vi "Menu.vi"() -> ()   [LabVIEW 2021]
panel:
  out "error out":errorcluster
  in  "error in":errorcluster
  out "String":string
  in  "Exit":bool
  out "Access":bool
  in  "Cluster":T1
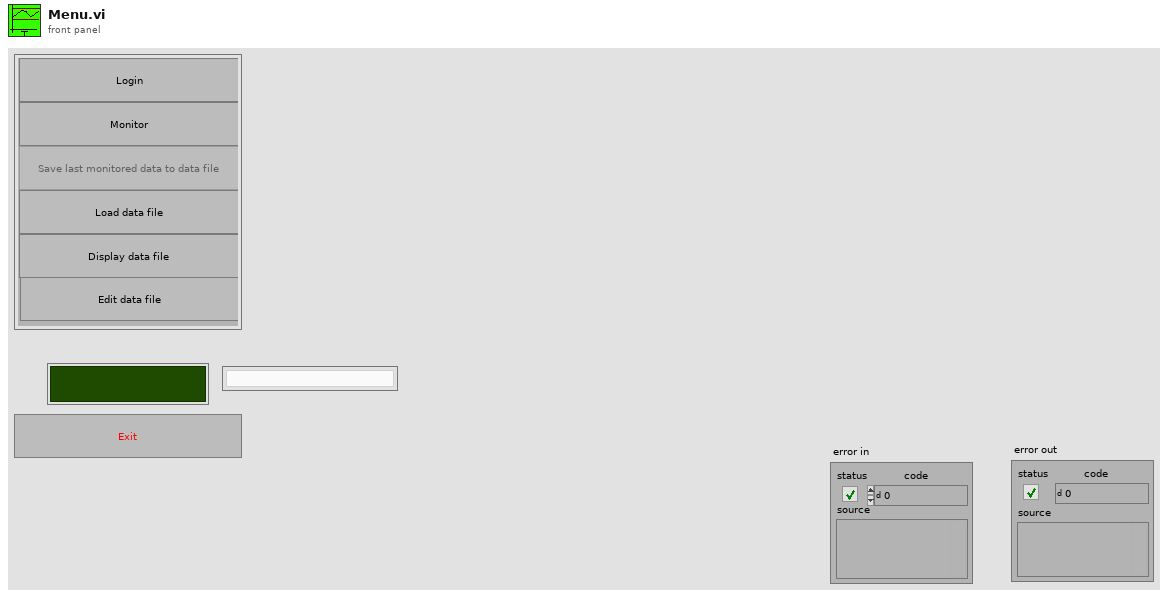
[diagram p1: front panel]
types:
  T1 = cluster{"Login button":bool, "Monitor button":bool, "Save data button":bool, "Load data button":bool, "Display data button":bool, "Edit Data File":bool}
  T2 = enum8{"Enabled", "Disabled", "Disabled and Grayed Out"}
  T3 = cluster{"User Name output":string, "Time/Date":timestamp, "Datos Finales":cluster{"Temp.Max":dbl, "Temp.Actual":dbl, "Temp.Min":dbl}[]}
  T4 = cluster{"User Name":string, "Time/Date":timestamp, "Datos Finales":cluster{"Temp.Max":dbl, "Temp.Actual":dbl, "Temp.Min":dbl}[]}
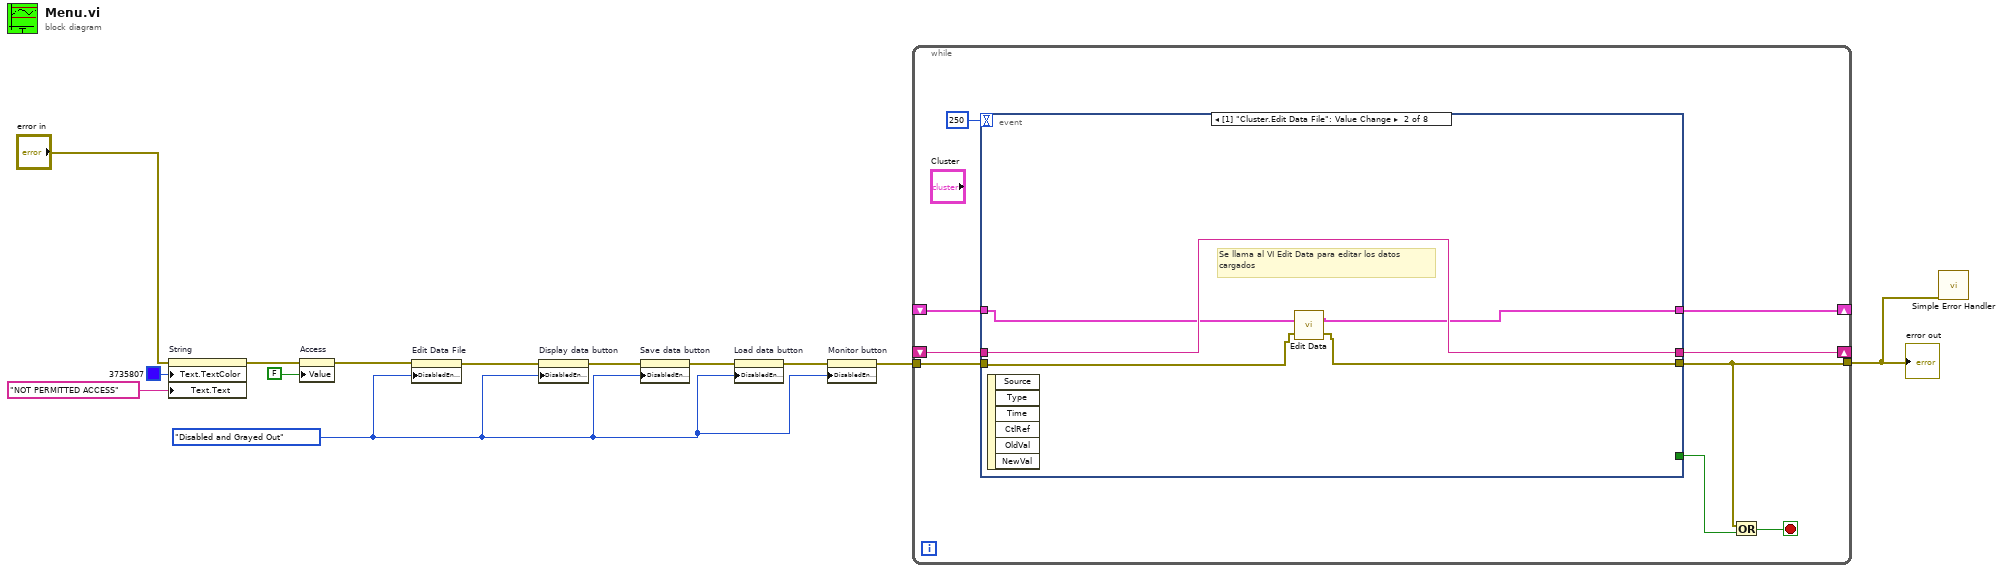
[diagram p0: block diagram]
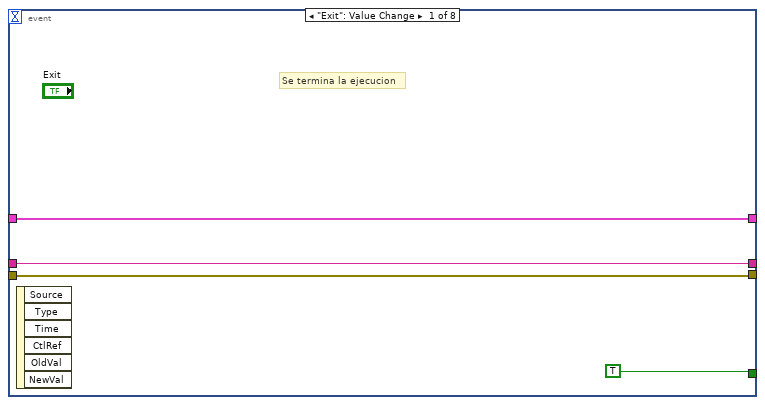
[diagram p2: hidden frame]
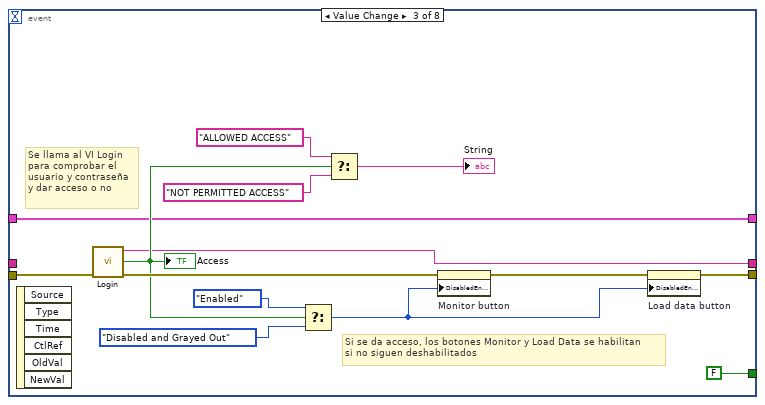
[diagram p3: hidden frame]
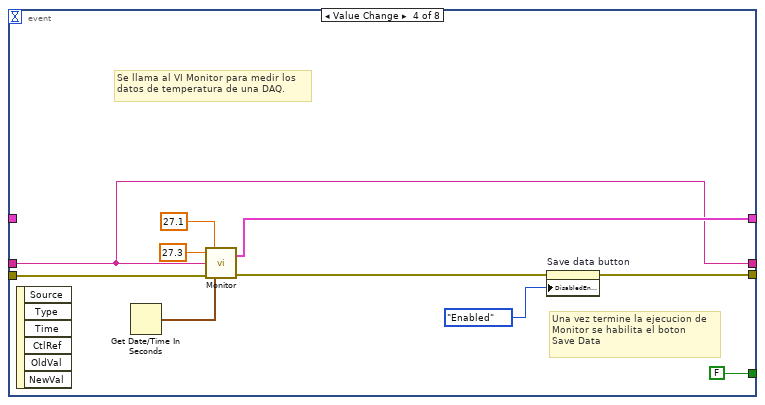
[diagram p4: hidden frame]
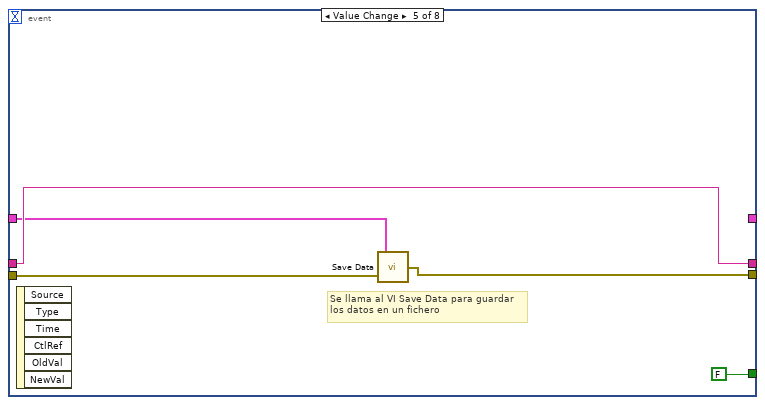
[diagram p5: hidden frame]
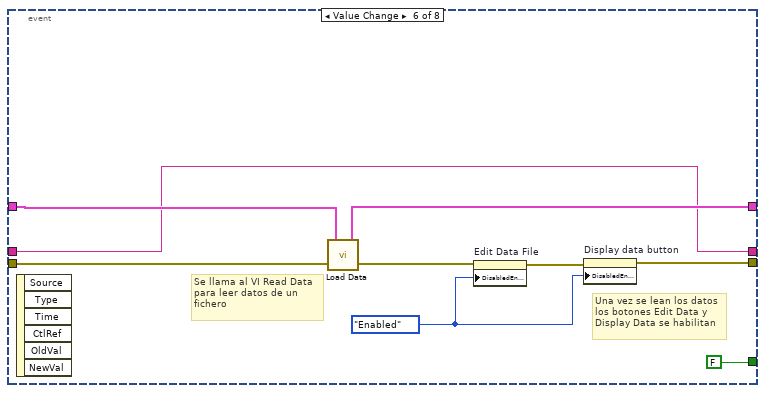
[diagram p6: hidden frame]
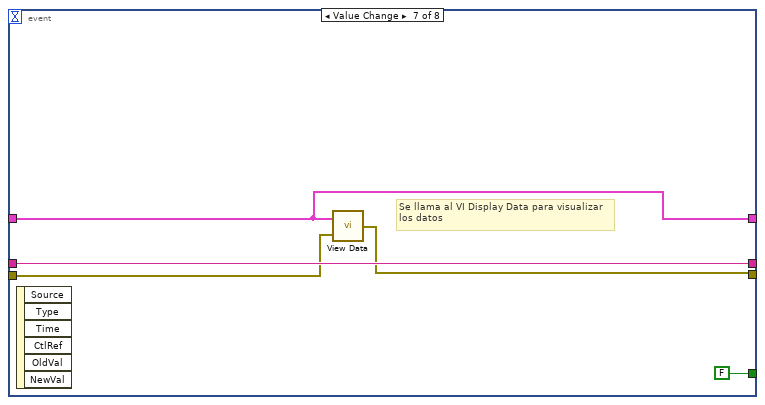
[diagram p7: hidden frame]
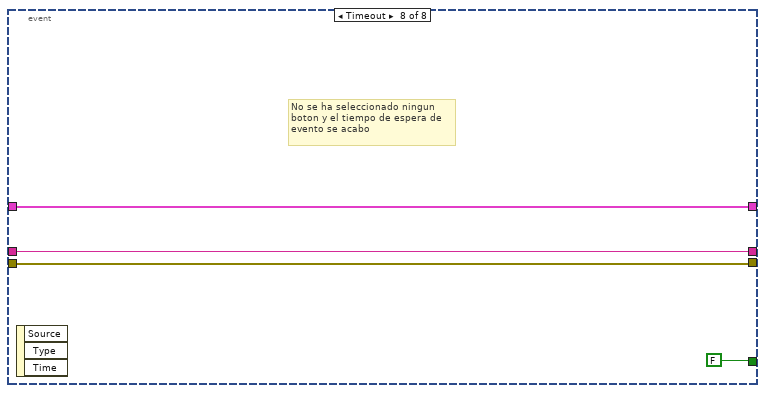
[diagram p8: hidden frame]
diagram:
  w1 = T2."Disabled and Grayed Out" ("Disabled")
  n1 = property on="String" class="Str"(error in="error in", "Text.TextColor"=u32 3735807 ("Text.Text Colors:Text Color"), "Text.Text"="NOT PERMITTED ACCESS") -> (error out=w7:errorcluster)  [unwired: 1 in, 1 out]
  n2 = property on="Access" class="Bool (strict)"(error in=w7, "Value"=FALSE ("Access")) -> (error out=w3:errorcluster)  [unwired: 1 in, 1 out]
  n3 = property on="Edit Data File" class="Bool"(error in=w3, "DisabledEnum"=w1) -> (error out=w2:errorcluster)  [unwired: 1 in, 1 out]
  n4 = property on="Display data button" class="Bool"(error in=w2, "DisabledEnum"=w1) -> (error out=w13:errorcluster)  [unwired: 1 in, 1 out]
  n5 = property on="Save data button" class="Bool"(error in=w13, "DisabledEnum"=w1) -> (error out=w12:errorcluster)  [unwired: 1 in, 1 out]
  n6 = property on="Load data button" class="Bool"(error in=w12, "DisabledEnum"=w1) -> (error out=w10:errorcluster)  [unwired: 1 in, 1 out]
  n7 = property on="Monitor button" class="Bool"(error in=w10, "DisabledEnum"=w1) -> (error out=w11:errorcluster)  [unwired: 1 in, 1 out]
  n8 = while {
    tunnel: [w20] -> w4
    tunnel: w11 -> [w21]
    shift-right: [w17] -> _
    shift-left: _ -> [w16]
    shift-right: [w15] -> _
    shift-left: _ -> [w14]
    stop <- w18 stop-if-true
    n9 = event shown="[1] \"Cluster.Edit Data File\": Value Change" {
      selector: _ -> [_ _ _ _ _ _ _ _]
      dyn-events: _ -> [_ _ _ _ _ _ _ _]
      timeout: 250 -> [_ _ _ _ _ _ _ _]
      tunnel: [TRUE _ FALSE FALSE FALSE FALSE FALSE FALSE] -> w19
      tunnel: [w25 w27 w42 w54 w57 w68 w71 w78] -> w20
      tunnel: w21 -> [w25 w29 w44 w50 w56 w66 w72 w78]
      tunnel: [w23 w31 w34 w46 w59 w64 w73 w76] -> w17
      tunnel: w16 -> [w23 w31 _ w46 w59 w64 w73 w76]
      tunnel: [w24 w28 w32 w47 _ w65 w70 w75] -> w15
      tunnel: w14 -> [w24 w30 w32 _ w58 w67 w70 w75]
      event "Exit": Value Change {
        # "Se termina la ejecucion"
        n10 = event-data() -> ()  [unwired: 1 in, 6 out]
      }
      event "Cluster.Edit Data File": Value Change {
        # "Se llama al VI Edit Data para editar los datos\ncargados"
        n11 = event-data() -> ()  [unwired: 1 in, 6 out]
        n12 = call "Edit Data.vi"("error in (no error)"=w29, "History Data input"=w30) -> ("error out"=w27:errorcluster, "History Data output"=w28:T3)
      }
      event "Cluster.Login button": Value Change {
        # "Si se da acceso, los botones Monitor y Load Data se habilitan\nsi no siguen deshabilitados"
        # "Se llama al VI Login \npara comprobar el \nusuario y contraseña\ny dar acceso o no"
        n13 = event-data() -> ()  [unwired: 1 in, 6 out]
        n14 = call "Login.vi"("error in (no error)"=w44) -> ("error out"=w43:errorcluster, "Access"=w35:bool, "User"=w34:string)  [unwired: 4 in]
        "Access" <- w35
        n15 = Select(t=T2."Enabled" ("Disabled"), s=w35, f=T2."Disabled and Grayed Out" ("Disabled")) -> (s? t:f=w39:T2)
        n16 = Select(t="ALLOWED ACCESS", s=w35, f="NOT PERMITTED ACCESS") -> (s? t:f=→"String":string)
        n17 = property on="Monitor button" class="Bool"(error in=w43, "DisabledEnum"=w39) -> (error out=w33:errorcluster)  [unwired: 1 in, 1 out]
        n18 = property on="Load data button" class="Bool"(error in=w33, "DisabledEnum"=w39) -> (error out=w42:errorcluster)  [unwired: 1 in, 1 out]
      }
      event "Cluster.Monitor button": Value Change {
        # "Una vez termine la ejecucion de\nMonitor se habilita el boton\nSave Data"
        # "Se llama al VI Monitor para medir los\ndatos de temperatura de una DAQ."
        n19 = event-data() -> ()  [unwired: 1 in, 6 out]
        n20 = Get Date/Time In Seconds() -> (seconds since 1Jan1904=w49:timestamp)
        n21 = call "Monitor.vi"("Temp.Max"=27.3, "Temp.Min"=27.1, "User name input"=w46, "error in (no error)"=w50, "Time/Date"=w49) -> ("History Data"=w47:T3, "error out"=w48:errorcluster)
        n22 = property on="Save data button" class="Bool"(error in=w48, "DisabledEnum"=T2."Enabled" ("Disabled")) -> (error out=w54:errorcluster)  [unwired: 1 in, 1 out]
      }
      event "Cluster.Save data button": Value Change {
        # "Se llama al VI Save Data para guardar \nlos datos en un fichero"
        n23 = event-data() -> ()  [unwired: 1 in, 6 out]
        n24 = call "Save Data.vi"("error in (no error)"=w56, "History Data"=w58) -> ("error out"=w57:errorcluster)
      }
      event "Cluster.Load data button": Value Change {
        w61 = T2."Enabled" ("Disabled")
        # "Una vez se lean los datos\nlos botones Edit Data y\nDisplay Data se habilitan"
        # "Se llama al VI Read Data \npara leer datos de un\nfichero"
        n25 = event-data() -> ()  [unwired: 1 in, 6 out]
        n26 = call "Load Data.vi"("error in (no error)"=w66, "History Data"=w67) -> ("error out"=w63:errorcluster, "History Data Output"=w65:T4)
        n27 = property on="Edit Data File" class="Bool"(error in=w63, "DisabledEnum"=w61) -> (error out=w62:errorcluster)  [unwired: 1 in, 1 out]
        n28 = property on="Display data button" class="Bool"(error in=w62, "DisabledEnum"=w61) -> (error out=w68:errorcluster)  [unwired: 1 in, 1 out]
      }
      event "Cluster.Display data button": Value Change {
        # "Se llama al VI Display Data para visualizar\nlos datos"
        n29 = event-data() -> ()  [unwired: 1 in, 6 out]
        n30 = call "View Data.vi"("error in (no error)"=w72, "Historic Data Input"=w70) -> ("error out"=w71:errorcluster)
      }
      event Timeout {
        # "No se ha seleccionado ningun\nboton y el tiempo de espera de\nevento se acabo"
        n31 = event-data() -> ()  [unwired: 1 in, 3 out]
      }
    }
    n32 = Or(x=w20, y=w19) -> (x .or. y?=w18:bool)
  }
  "error out" <- w4
  n33 = call <vilib>:"Simple Error Handler.vi"("error in (no error)"=w4) -> ()  [unwired: 4 in, 5 out]
